vi "isComplete.vi"(8 "error in (no error)":errorcluster, 11 "Mission in":refnum<class "Idle.lvclass">) -> (0 "error out":errorcluster, 2 "Mission Complete?":bool, 3 "Mission out":refnum<class "Idle.lvclass">)   [LabVIEW 2011, in "Idle.lvclass"]
doc: "Determine whether or not a mission is complete.\n\nNote: This is a dynamic dispatch method of GenericMission. The correct method will be called based on the run-time class of this object, a child class of GenericMission.\n\nAuthor: Jared Kirschner"
uses:
  Idle.lvclass
  Idle.lvclass/Idle.ctl
  2 Globals/2 Global.vi
  MissionQueue/MissionQueue.lvclass
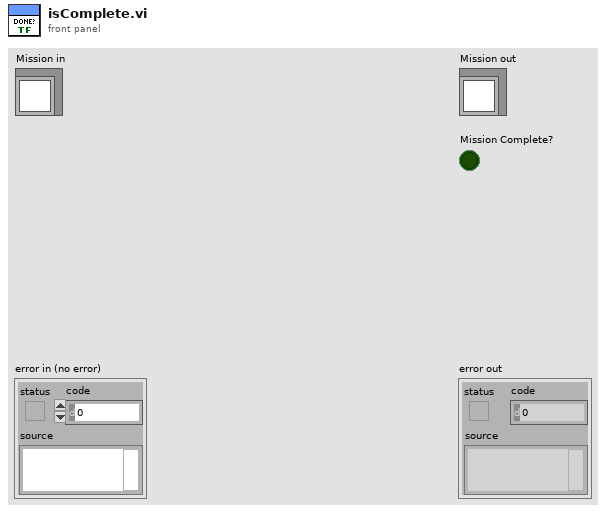
[diagram p1: front panel]
types:
  T1 = typedef "Waypoints List.ctl" = refnum<class "Waypoint.lvclass">[]
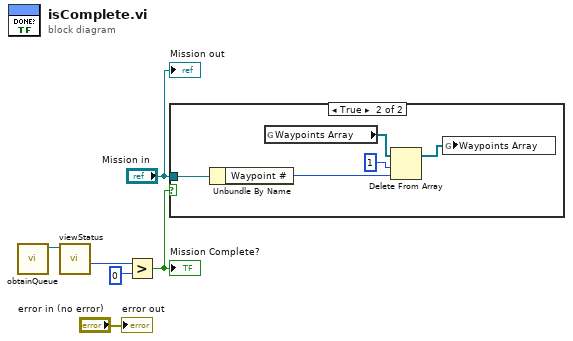
[diagram p0: block diagram]
diagram:
  n1 = call "obtainQueue.vi"() -> ("MissionQueue.lvclass"=w5:refnum<class "MissionQueue.lvclass">)  [unwired: 10 in, 1 out]
  n2 = call "viewStatus.vi"("MissionQueue in"=w5) -> ("Queue length"=w4:i32)  [unwired: 7 in, 3 out]
  n3 = Greater?(x=w4, y=0) -> (0:w1:bool)
  "Mission Complete?" <- w1
  n4 = case shown="True" w1 {
    tunnel: "Mission in" -> [_ w8]
    frame False {
    }
    frame True {
      n5 = Unbundle By Name(w8) -> ("Waypoint #"=w9:i32)
      n6 = global read "2 Global.vi" "Waypoints Array"() -> (w11:T1)
      n7 = Delete From Array(array=w11, length=1, index=w9) -> (array with subset deleted=w7:T1)  [unwired: 1 out]
      n8 = global write "2 Global.vi" "Waypoints Array"(w7) -> ()
    }
  }
  "error out" <- "error in (no error)"
  "Mission out" <- "Mission in"
